vi "get_project_path.vi"(8 "error in (no error)":errorcluster) -> (0 "error out":errorcluster, 2 "helioscan path":path)   [LabVIEW 2010]
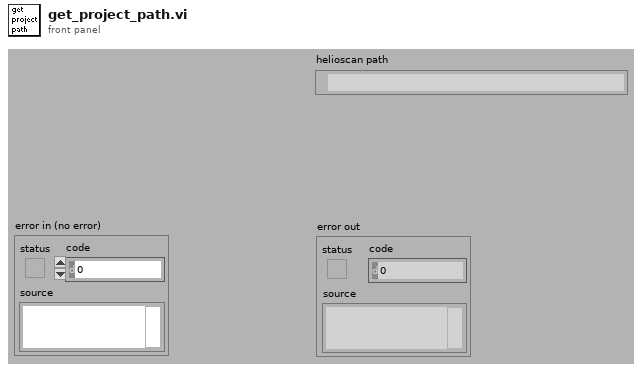
[diagram p1: front panel]
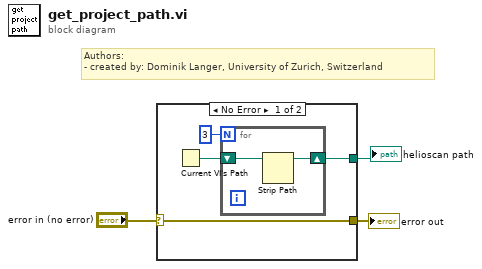
[diagram p0: block diagram]
diagram:
  # "Authors: \n- created by: Dominik Langer, University of Zurich, Switzerland"
  n1 = case shown="No Error" "error in (no error)" {
    selector: "error in (no error)" -> [w6 w10]
    tunnel: [w5 _] -> w3
    tunnel: [w6 w10] -> w1
    frame No Error {
      n2 = Current VI's Path() -> (path=w7:path)
      n3 = for {
        N: 3 -> [_]
        shift-right: [w8] -> w5
        shift-left: w7 -> [w9]
        n4 = Strip Path(path=w9) -> (stripped path=w8:path)  [unwired: 1 out]
      }
    }
    frame Error {
    }
  }
  "helioscan path" <- w3
  "error out" <- w1
